vi "Util_Convert Hex String to String.vi"(4 "Hex String":string) -> (1 "String":string)   [LabVIEW 2014]
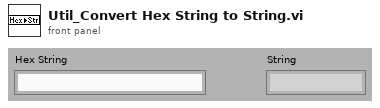
[diagram p1: front panel]
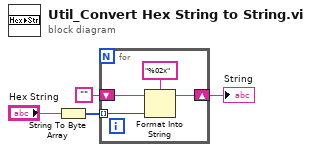
[diagram p0: block diagram]
diagram:
  n1 = String To Byte Array(string="Hex String") -> (unsigned byte array=w3:u8[])
  n2 = for {
    tunnel: w3 -> [w8] mode=indexing
    shift-right: [w6] -> w2
    shift-left: "" -> [w7]
    n3 = Format Into String(format string="%02x", initial string=w7, w8) -> (resulting string=w6:string)  [unwired: 1 in, 1 out]
  }
  "String" <- w2
